vi "Configure.vi"(0 "SG Path Power Meter Accessor in":refnum<class "SG Path Accessor.lvclass">, 5 "frequency":dbl=50000000.0, 11 "error in (no error)":errorcluster) -> (4 "SG Path Power Meter Accessor out":refnum<class "SG Path Accessor.lvclass">, 15 "error out":errorcluster)   [LabVIEW 2023, in "NI-568x RF Power Meter.lvlib" / "SG Path Accessor.lvclass"]
uses:
  SG Path Accessor.lvclass
  Power Meter/Power Meter.lvclass
  Power Meter/Power Meter.lvclass/Power Meter.ctl
  Power Meter/Properties/Read Resource Name.vi
  Instruments/Power Meter/Power Meter Factory/Power Meter Factory.lvclass
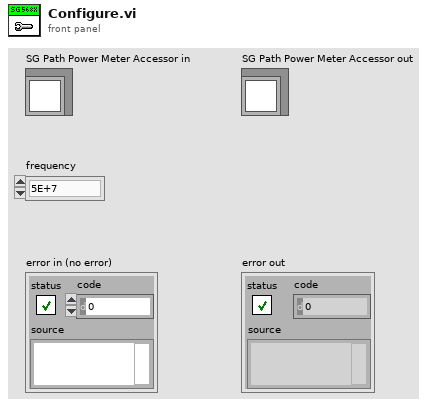
[diagram p1: front panel]
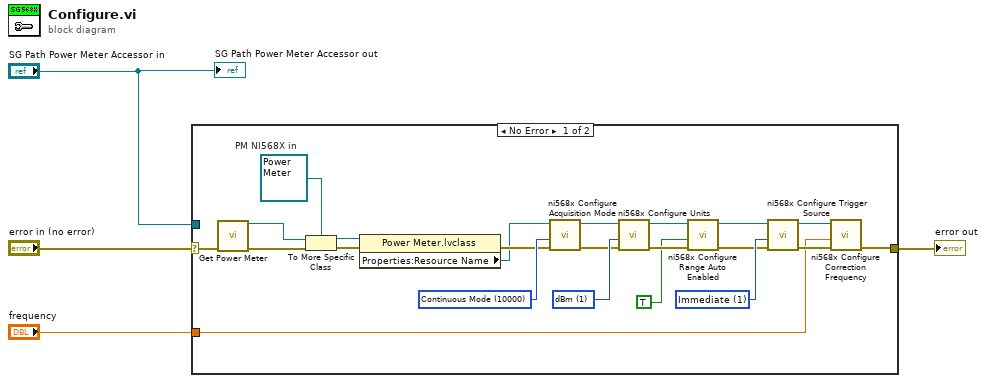
[diagram p0: block diagram]
diagram:
  n1 = case shown="No Error" "error in (no error)" {
    selector: "error in (no error)" -> [w26 w27]
    tunnel: [w5 w27] -> w4
    tunnel: "SG Path Power Meter Accessor in" -> [_ _]
    tunnel: "frequency" -> [w14 _]
    frame No Error {
      w12 = refnum<class "Power Meter.lvclass"> refnum  # PM NI568X in
      w20 = 10000 items=["Continuous Mode"=10000, "Time Slot Mode"=20000, "Scope Mode"=30000] ("mode")
      w22 = 1 items=["Immediate"=1, "External"=2, "Internal"=3, "Software"=4] ("trigger source")
      w25 = 1 items=["dBm"=1, "Watts"=4, "mWatts"=1001, "uWatts"=1002] ("units")
      n2 = call "Get Power Meter.vi"("error in (no error)"=w26) -> ("Power Meter Base out"=w11:refnum<class "Power Meter Base.lvclass">, "error out"=w13:errorcluster)  [unwired: 13 in]
      n3 = To More Specific Class(target class=w12, reference=w11, error in=w13) -> (specific class reference=w16:refnum<class "Power Meter.lvclass">, error out=w18:errorcluster)
      n4 = property class="Power Meter.lvclass"(reference=w16, error in=w18) -> (error out=w17:errorcluster, "Properties:Resource Name"=w10:refnum<k15>)  [unwired: 1 out]
      n5 = call <instrlib>:"ni568x Configure Acquisition Mode.vi"("instrument handle"=w10, "mode"=w20, "error in"=w17) -> ("instrument handle out"=w9:refnum<k15>, "error out"=w19:errorcluster)  [unwired: 6 in]
      n6 = call <instrlib>:"ni568x Configure Units.vi"("error in"=w19, "units"=w25, "instrument handle"=w9) -> ("error out"=w24:errorcluster, "instrument handle out"=w8:refnum<k15>)  [unwired: 7 in]
      n7 = call <instrlib>:"ni568x Configure Range Auto Enabled.vi"("error in"=w24, "range auto enabled"=TRUE, "instrument handle"=w8) -> ("error out"=w21:errorcluster, "instrument handle out"=w7:refnum<k15>)  [unwired: 7 in]
      n8 = call <instrlib>:"ni568x Configure Trigger Source.vi"("error in"=w21, "trigger source"=w22, "instrument handle"=w7) -> ("error out"=w15:errorcluster, "instrument handle out"=w6:refnum<k15>)  [unwired: 7 in]
      n9 = call <instrlib>:"ni568x Configure Correction Frequency.vi"("error in"=w15, "frequency"=w14, "instrument handle"=w6) -> ("error out"=w5:errorcluster)  [unwired: 7 in, 1 out]
    }
    frame Error {
    }
  }
  "error out" <- w4
  "SG Path Power Meter Accessor out" <- "SG Path Power Meter Accessor in"
